vi "TB-Slack Figure.vi"(0 "Log":T1, 1 "XYGraph in":refnum<vi>) -> (15 "error out":errorcluster)   [LabVIEW 2020]
uses:
  Typedefs/TB-Log.ctl
  Typedefs/TB-Slack State.ctl
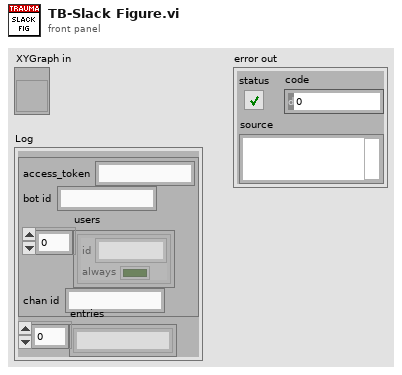
[diagram p1: front panel]
types:
  T1 = typedef "TB-Log.ctl" = cluster{"Slack":T2, "entries":string[]}
  T2 = typedef "TB-Slack State.ctl" = cluster{"access_token":string, "bot id":string, "users":cluster{"id":string, "always":bool}[], "chan id":string}
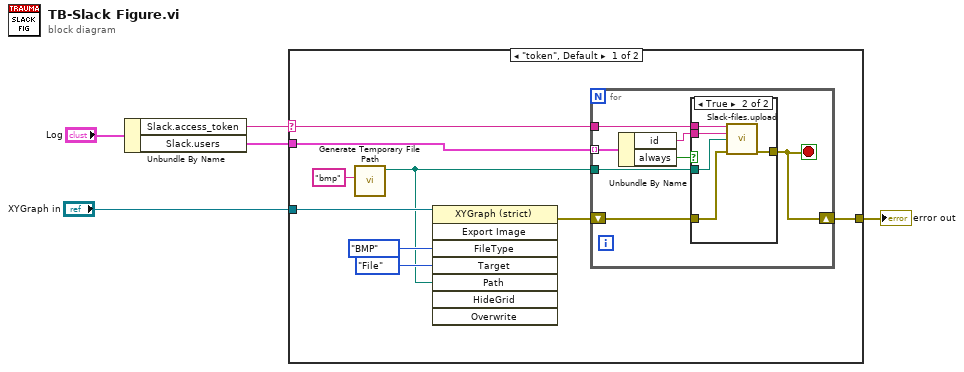
[diagram p0: block diagram]
diagram:
  n1 = Unbundle By Name("Log") -> ("Slack.access_token"=w4:string, "Slack.users"=w3:cluster{"id":string, "always":bool}[])
  n2 = case shown="\"token\", Default" w4 {
    selector: w4 -> [w14 _]
    tunnel: w3 -> [w13 _]
    tunnel: [w12 _] -> w2
    tunnel: "XYGraph in" -> [w11 _]
    frame "token", Default {
      n3 = call <vilib>:"Generate Temporary File Path.vi"("Temporary File Extension (tmp)"="bmp") -> ("Unique Temporary File Path"=w7:path)  [unwired: 9 in, 1 out]
      n4 = invoke class="XYGraph (strict)" method="Export Image"(reference=w11, "FileType"=enum32{"BMP", "EPS", "EMF", "PICT"}."BMP" ("File Type"), "Target"=enum32{"File", "Clipboard"}."File", "Path"=w7) -> (error out=w8:errorcluster)  [unwired: 4 in, 7 out]
      n5 = for {
        tunnel: w14 -> [w21]
        tunnel: w13 -> [w17] mode=indexing
        shift-right: [w20] -> w12
        shift-left: w8 -> [w19]
        tunnel: w7 -> [w18]
        stop <- w20 stop-if-true
        n6 = Unbundle By Name(w17) -> ("id"=w16:string, "always"=w15:bool)
        n7 = case shown="True" w15 {
          tunnel: w21 -> [_ w26]
          tunnel: [_ w25] -> w20
          tunnel: w19 -> [_ w24]
          tunnel: w18 -> [_ w23]
          tunnel: w16 -> [_ w22]
          frame False {
          }
          frame True {
            n8 = call "Slack-files.upload.vi"("token"=w26, "channels"=w22, "File"=w23, "error in (no error)"=w24) -> ("error out"=w25:errorcluster)  [unwired: 11 in]
          }
        }
      }
    }
    frame "" {
    }
  }
  "error out" <- w2
